vi "Initialize Resistor Interface.vi"(8 "error in (no error)":errorcluster, 10 "Color Box Refnum":refnum<vi>[](array[refnum]), 11 "Enum Refnum":refnum<vi>[](array[refnum])) -> (0 "error out":errorcluster)   [LabVIEW 2018]
uses:
  Digit--control.ctl
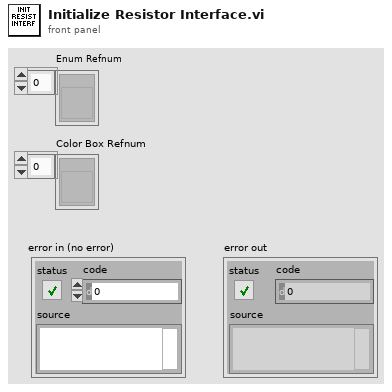
[diagram p1: front panel]
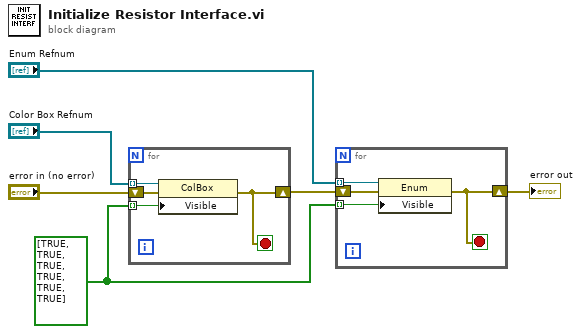
[diagram p0: block diagram]
diagram:
  w3 = bool[] [TRUE, TRUE, TRUE, TRUE, TRUE, TRUE]
  n1 = for {
    shift-right: [w7] -> w6
    shift-left: "error in (no error)" -> [w10]
    tunnel: w3 -> [w8] mode=indexing
    tunnel: "Color Box Refnum" -> [w9] mode=indexing
    stop <- w7 stop-if-true
    n2 = property class="ColBox"(reference=w9, error in=w10, "Visible"=w8) -> (error out=w7:errorcluster)  [unwired: 1 out]
  }
  n3 = for {
    shift-right: [w11] -> w4
    shift-left: w6 -> [w14]
    tunnel: w3 -> [w12] mode=indexing
    tunnel: "Enum Refnum" -> [w13] mode=indexing
    stop <- w11 stop-if-true
    n4 = property class="Enum"(reference=w13, error in=w14, "Visible"=w12) -> (error out=w11:errorcluster)  [unwired: 1 out]
  }
  "error out" <- w4
